vi "Acquire_Widefield.vi"() -> ()   [LabVIEW 2014]
uses:
  <vilib>/vision/Image Controls.llb/IMAQ Image.ctl
  <vilib>/userdefined/High Color/IMAQdx.ctl
  Widefield_globals.vi
  <vilib>/vision/NI_Vision_Development_Module.lvlib
  <vilib>/vision/driver/NI_Vision_Acquisition_Software.lvlib
panel:
  out "Camera Type":u16(ring)=1 items=["AVT Manta", "Hamamatsu Orca", "PhotonFocus GigE"]
  out "FOV size (um)":i32[](array[numeric])=[643, 394]
  in  "Spatial filter (um)":i32=100
  out "exposure (s)":dbl
  out "IMAQ session":T1 caption="Session Out"
  out "odor time":u32
  out "Waveform Graph":i32[](graph)
  out "frame gap":sgl
  out "frame times":i32[](array[numeric])
  out "error out":errorcluster
  out "LED settle":i32
  out "Control LED?":bool
  out "stim tag":string
  out "SF file":string
  out "One Bulb?":bool
  in  "Odor build up":dbl=5.0
  out "File Path":path
  out "SingleFrames":bool
  out "empty frame":dbl[][](array[numeric])
  out "Resolution":u32[](array[numeric])
  out "Experiment Sequence":dbl[][](array[numeric])
  out "settings":sgl[](array[numeric])
  out "Buff Img":T2
  out "IgorSAir":T2
  out "IgorOdor":T2
  out "IgorAir":T2
  out "RatioIm 2":dbl[][](graph)
  out "COString":string
  in  "Offset (32768 default)":u32=32768
  in  "Contrast \n(600000 default)":u32=600000
  out "FrameTime":u32
  in  "Pause":bool=TRUE
  out "ExpOrderRefnum":refnum<file>
  out "Subframes":u32
  out "DCSAir":dbl[][](array[numeric])
  out "DCOdor":dbl[][](array[numeric])
  out "DCAir":dbl[][](array[numeric])
  out "TiffRefnum":refnum<file>
  out "Indices":i32[](array[numeric])
  out "Frames SAir":u32
  out "RatioIm":dbl[][](graph)
  out "Odors:":u32
  out "StopAcq":bool
  in  "Stop":bool=TRUE
  out "Odor #":i32=50
  out "Repeats:":i32=1
  out "Repeat #":i32=1
  out "Frames Odor":u32
  out "Frames Air":u32
  out "Status":string
  out "Stimulus #":i32
  in  "start":bool=TRUE
  # "Filtered Ratio Image"
  # "Ratio Image"
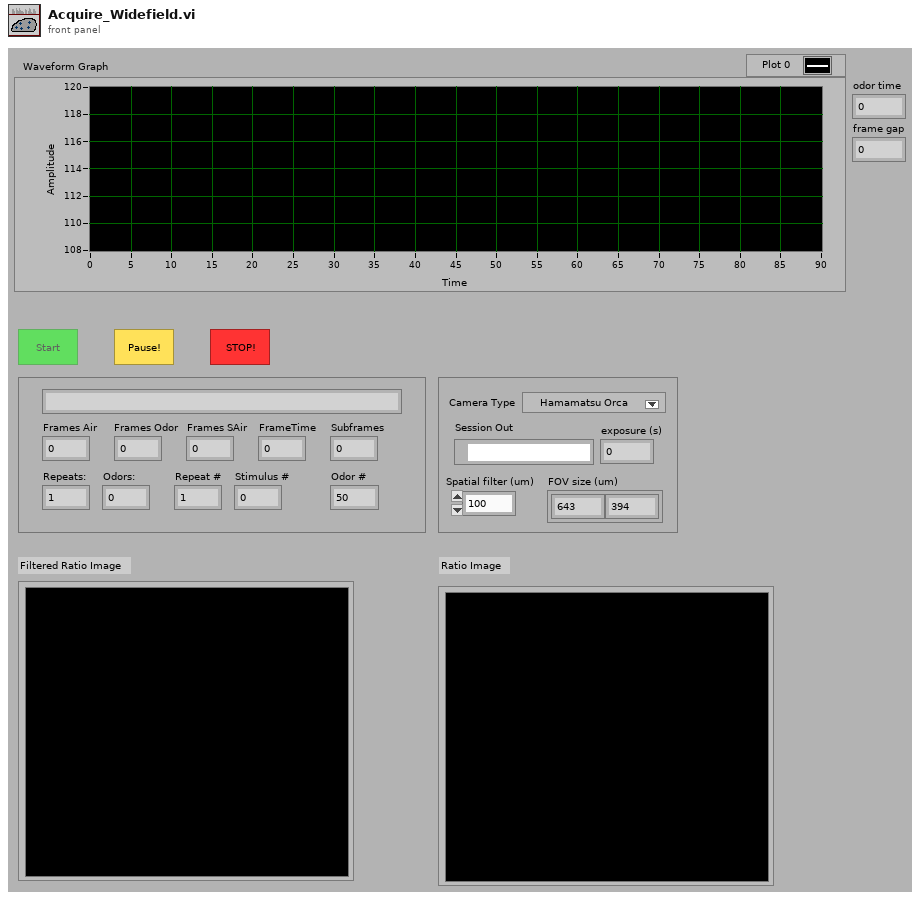
[diagram p1: front panel]
types:
  T1 = typedef "IMAQdx.ctl" = refnum<k21>
  T2 = typedef "IMAQ Image.ctl" = refnum<image>
  T3 = enum16{"open", "replace", "create", "open or create", "replace or create", "replace or create with confirmation"}
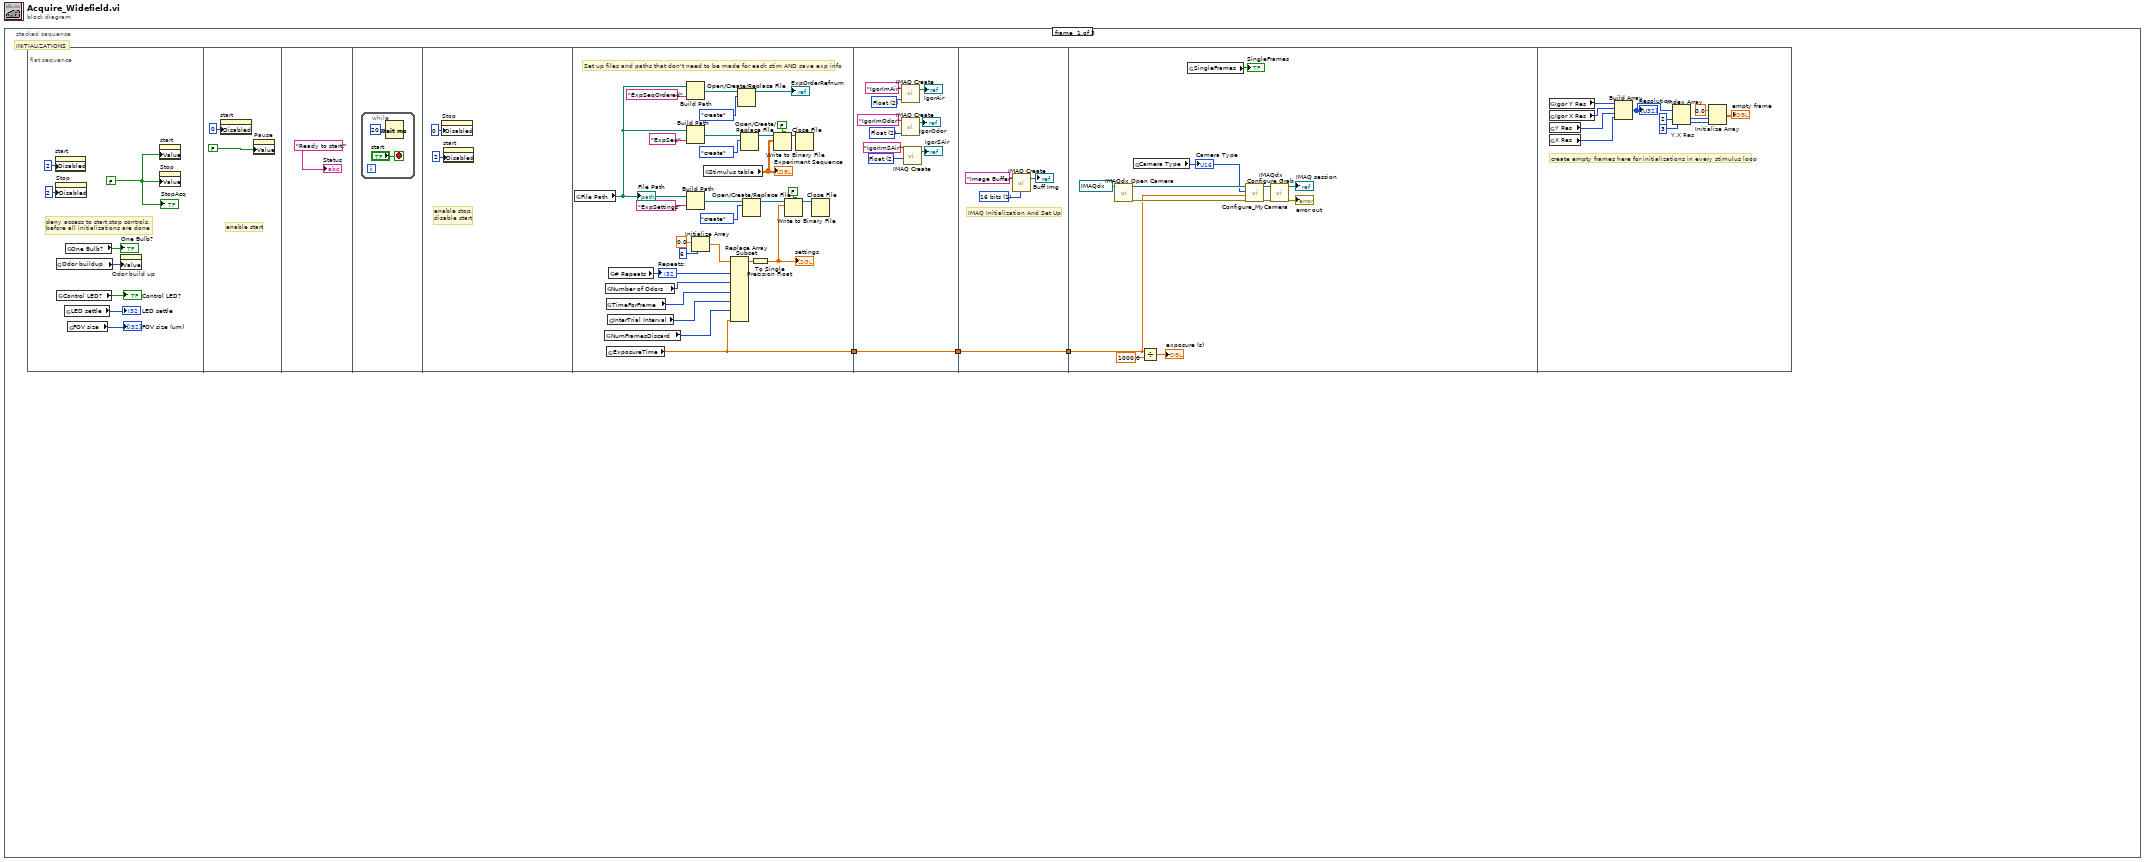
[diagram p0: block diagram]
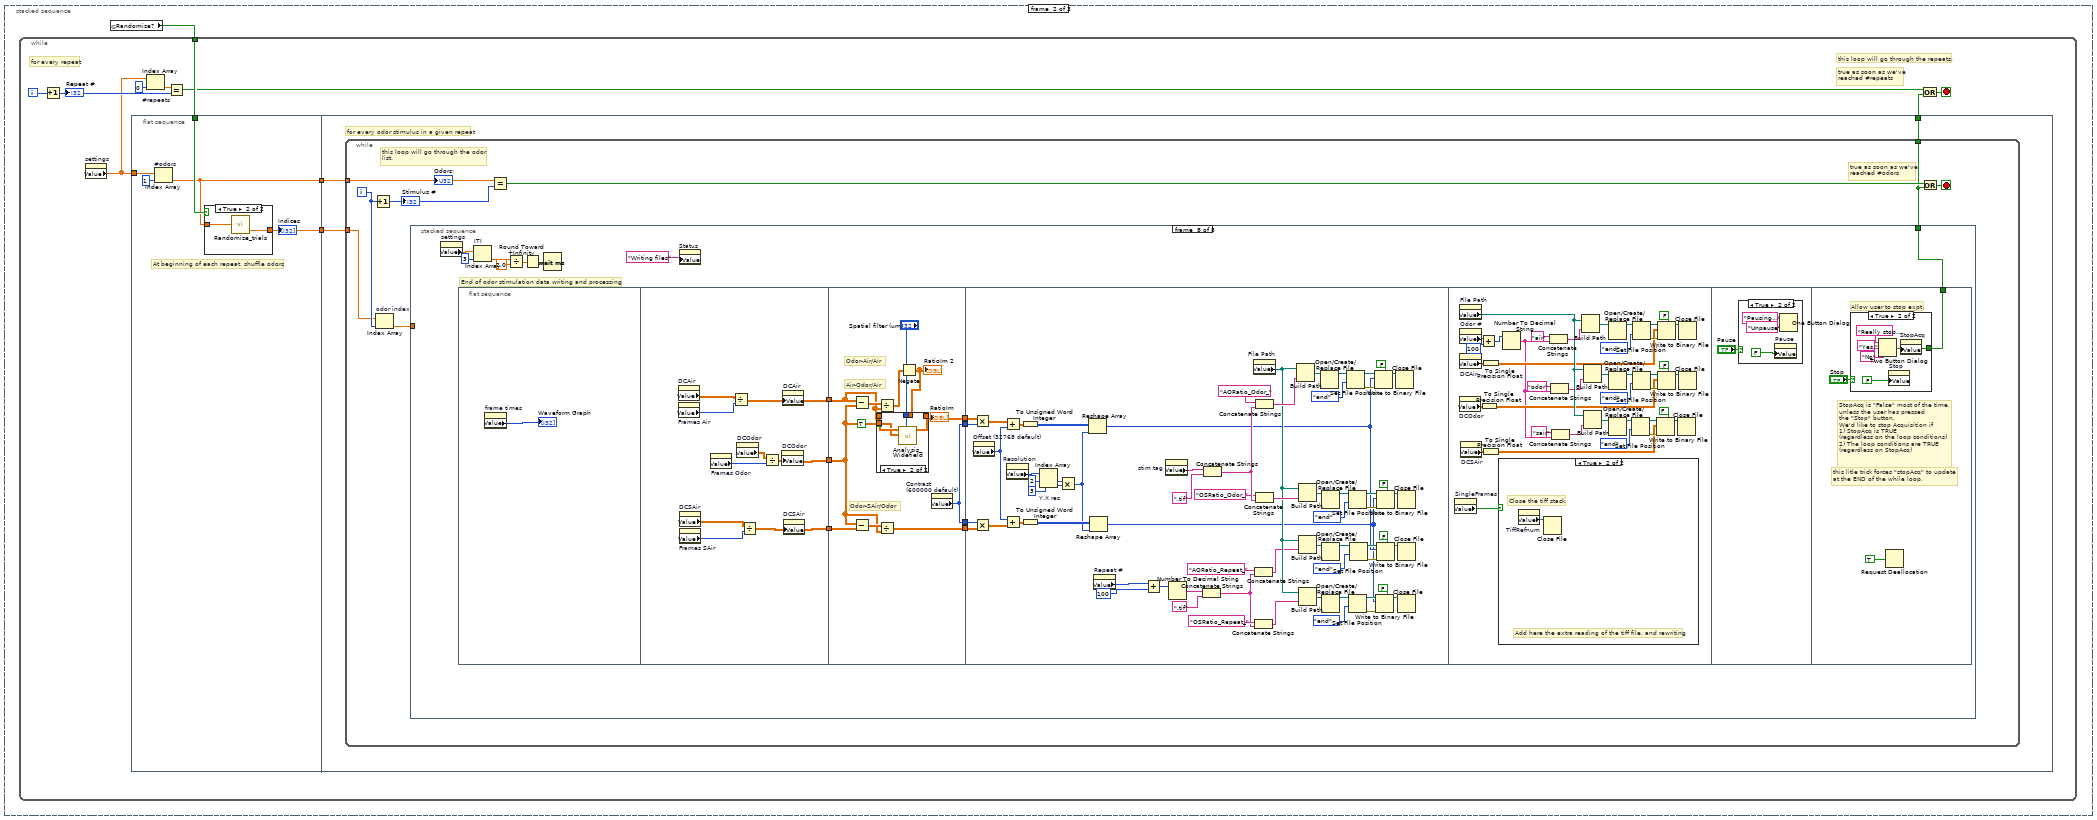
[diagram p2: hidden frame]
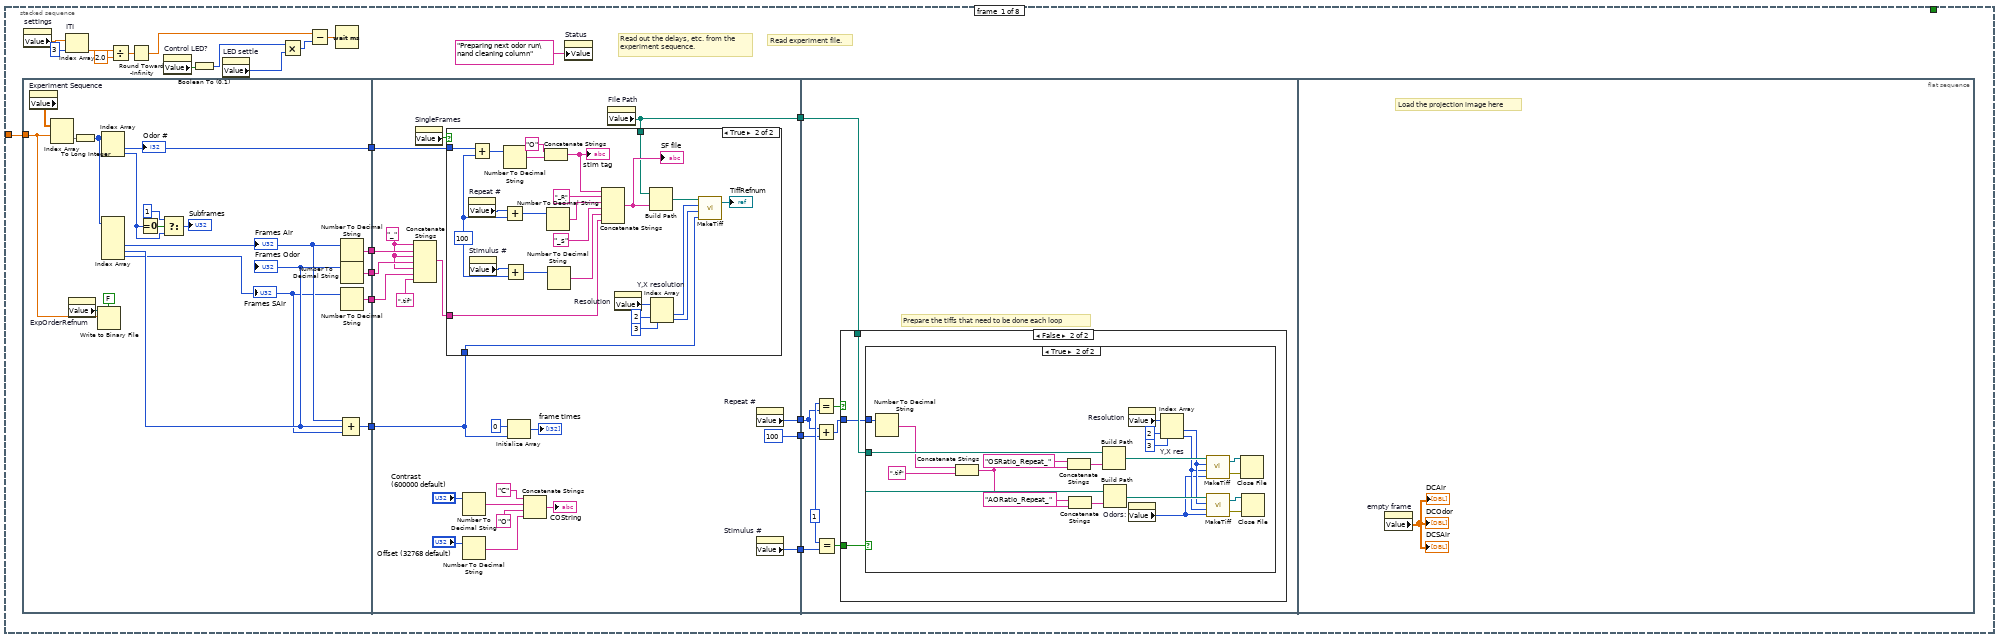
[diagram p4: hidden frame]
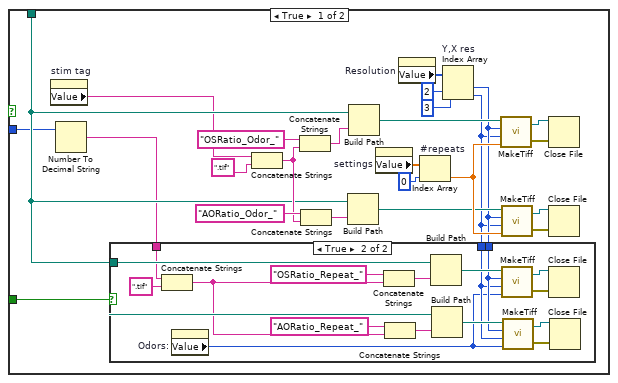
[diagram p6: hidden frame]
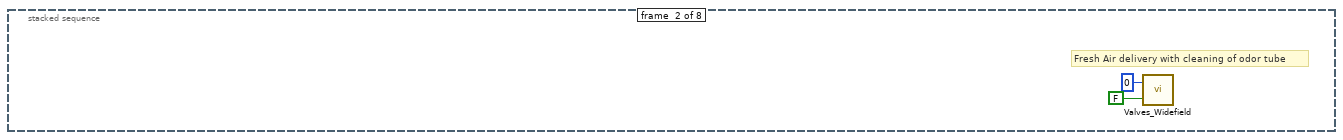
[diagram p9: hidden frame]
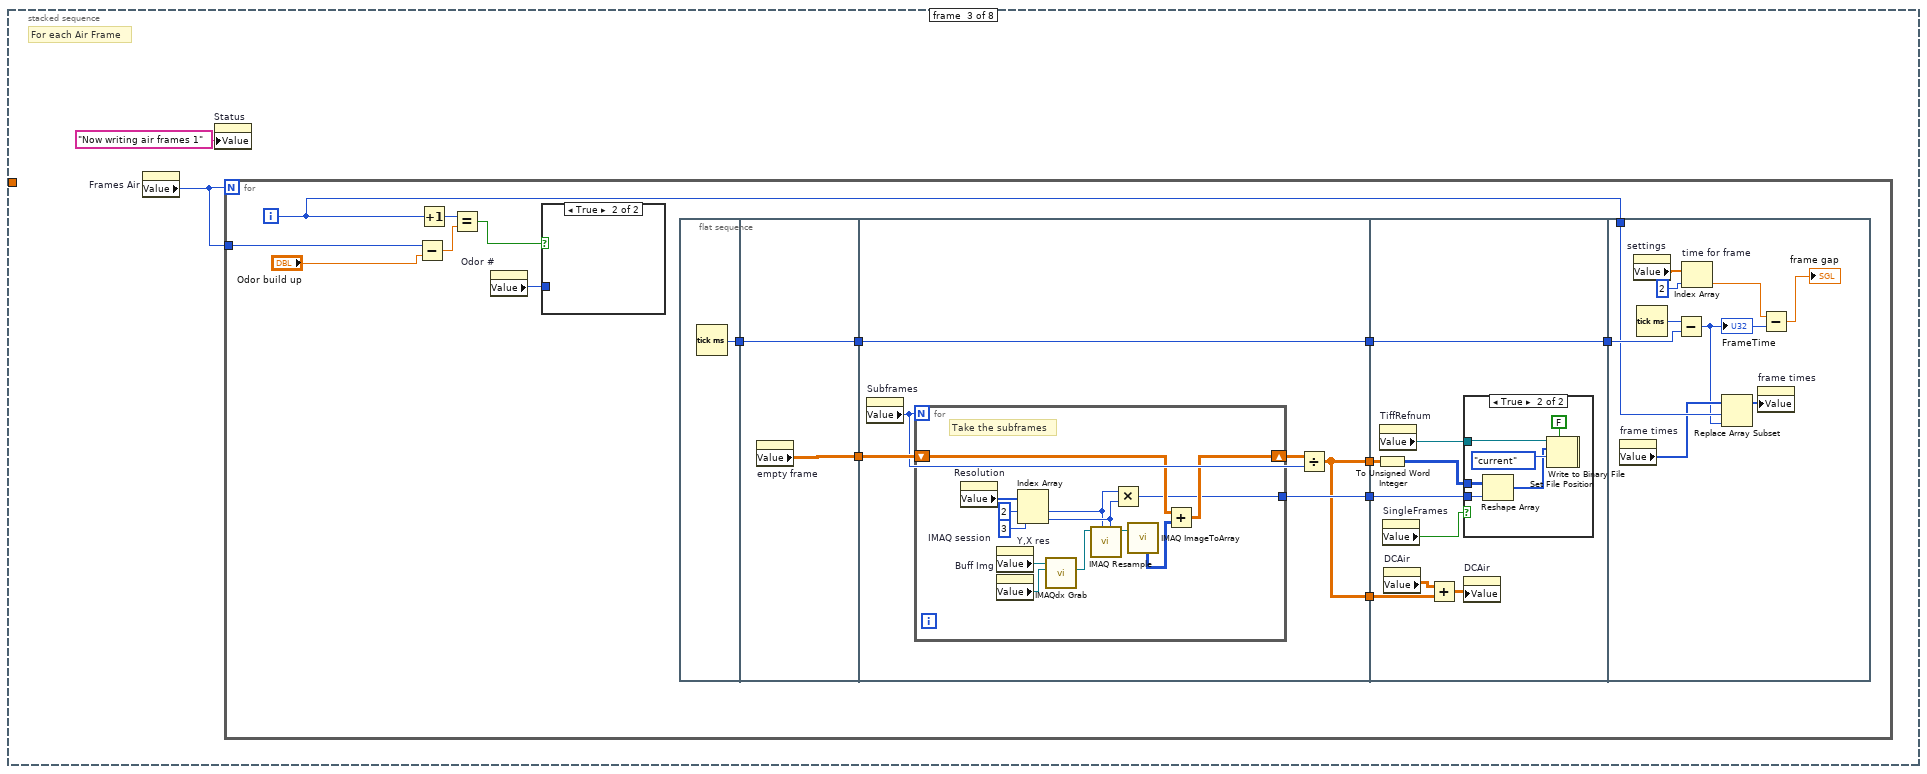
[diagram p10: hidden frame]
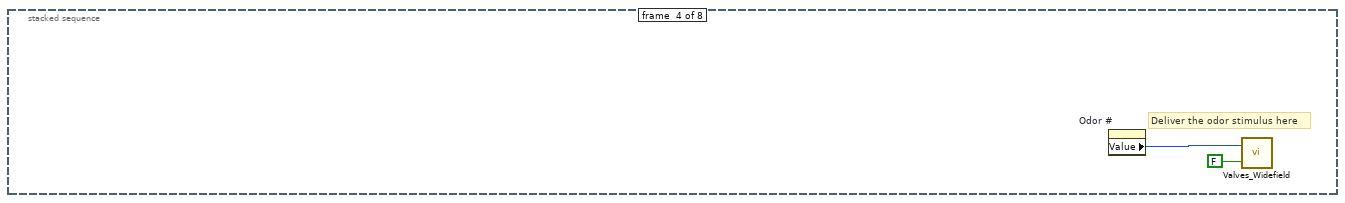
[diagram p13: hidden frame]
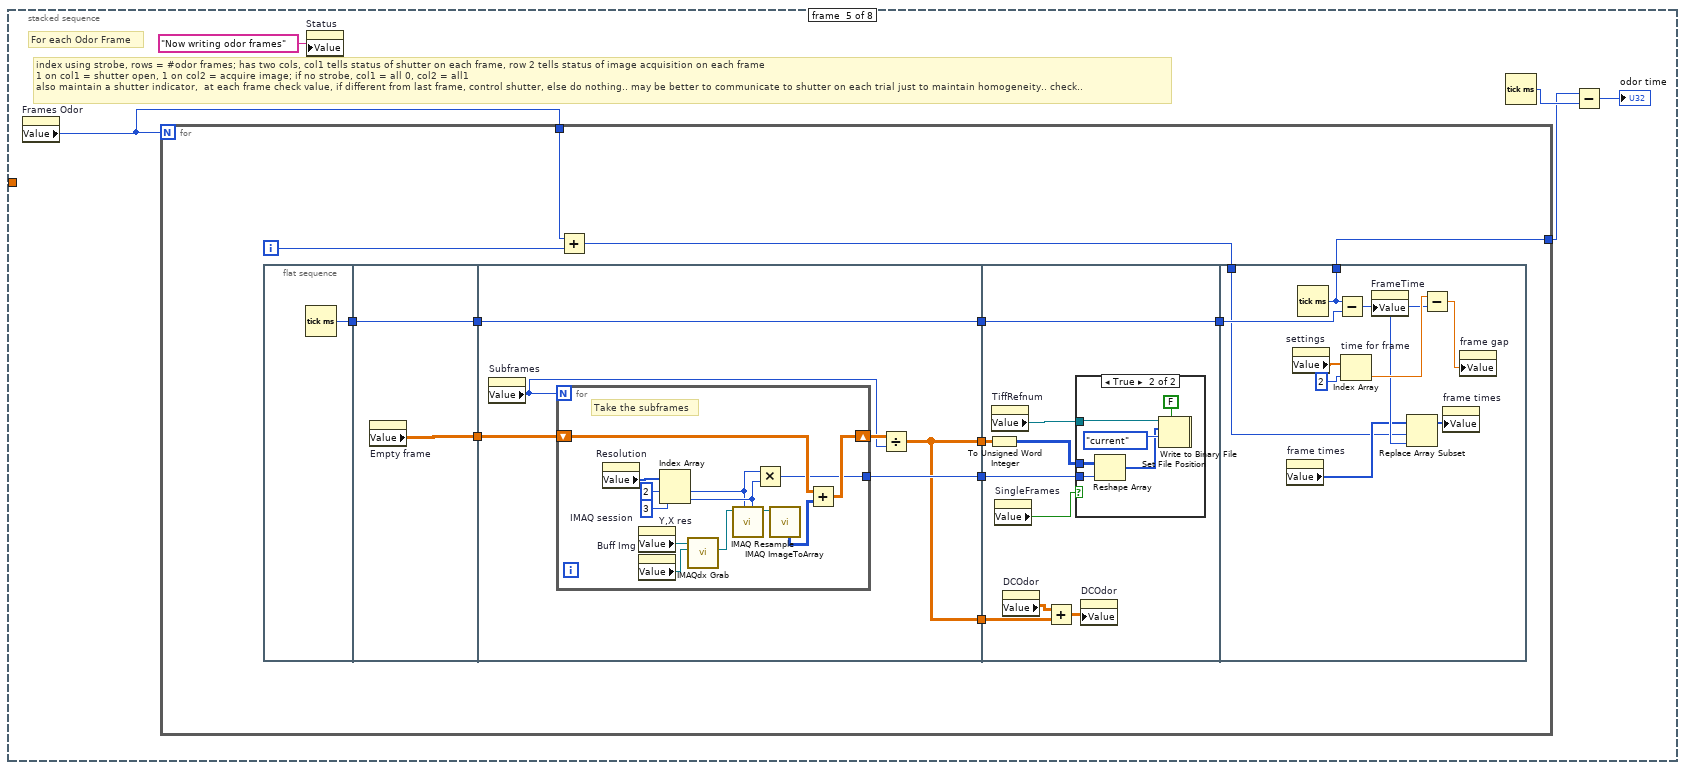
[diagram p14: hidden frame]
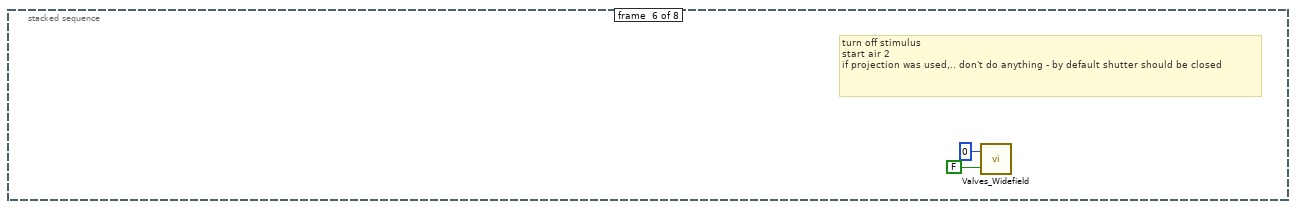
[diagram p16: hidden frame]
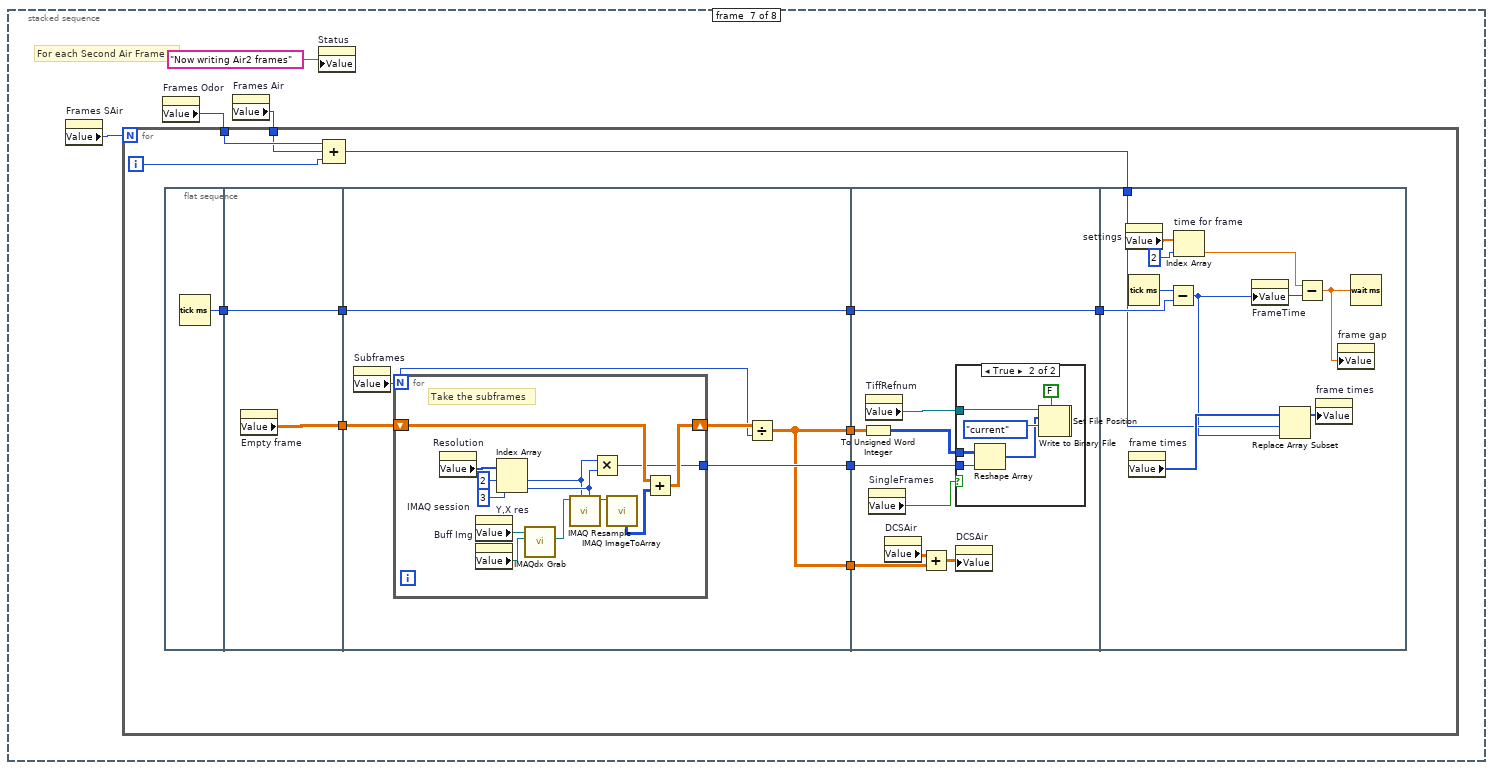
[diagram p17: hidden frame]
diagram:
  n1 = stacked-sequence {
    frame #0 {
      # "INITIALIZATIONS"
      n2 = flat-sequence {
        tunnel: [w20] -> w1
        tunnel: [w48] -> w2
        tunnel: w1 -> [w48]
        tunnel: [w58] -> w3
        tunnel: w2 -> [w58]
        tunnel: w3 -> [w65]
        frame #0 {
          w9 = FALSE ("Stop")
          # "deny access to start stop controls, \nbefore all initializations are done"
          n3 = property on="start" class="Bool (strict)"("Disabled"=u8 2) -> ()  [unwired: 2 in, 2 out]
          n4 = property on="Stop" class="Bool (strict)"("Disabled"=u8 2) -> ()  [unwired: 2 in, 2 out]
          n5 = global read "Widefield_globals.vi" "Odor buildup"() -> (w8:i32)
          n6 = global read "Widefield_globals.vi" "Control LED?"() -> (→"Control LED?":bool)
          n7 = global read "Widefield_globals.vi" "LED settle"() -> (→"LED settle":i32)
          n8 = global read "Widefield_globals.vi" "One Bulb?"() -> (→"One Bulb?":bool)
          n9 = global read "Widefield_globals.vi" "FOV size"() -> (→"FOV size (um)":i32[])
          n10 = property on="Odor build up" class="DigNum (strict)"("Value"=w8) -> ()  [unwired: 2 in, 2 out]
          n11 = property on="start" class="Bool (strict)"("Value"=w9) -> ()  [unwired: 2 in, 2 out]
          n12 = property on="Stop" class="Bool (strict)"("Value"=w9) -> ()  [unwired: 2 in, 2 out]
          "StopAcq" <- w9
        }
        frame #1 {
          # "enable start"
          n13 = property on="start" class="Bool (strict)"("Disabled"=u8 0) -> ()  [unwired: 2 in, 2 out]
          n14 = property on="Pause" class="Bool (strict)"("Value"=FALSE ("Pause")) -> ()  [unwired: 2 in, 2 out]
        }
        frame #2 {
          "Status" <- "Ready to start!" ("Status")
        }
        frame #3 {
          n15 = while {
            stop <- "start" stop-if-true
            n16 = Wait (ms)(milliseconds to wait=u32 20) -> ()  [unwired: 1 out]
          }
        }
        frame #4 {
          # "enable stop,\ndisable start"
          n17 = property on="Stop" class="Bool (strict)"("Disabled"=u8 0) -> ()  [unwired: 2 in, 2 out]
          n18 = property on="start" class="Bool (strict)"("Disabled"=u8 2) -> ()  [unwired: 2 in, 2 out]
        }
        frame #5 {
          # "Set up files and paths that don't need to be made for each stim AND save exp info"
          n19 = global read "Widefield_globals.vi" "File Path"() -> (w26:path)
          "File Path" <- w26
          n20 = global read "Widefield_globals.vi" "NumFramesDiscard"() -> (w21:i32)
          n21 = global read "Widefield_globals.vi" "Number of Odors"() -> (w23:u32)
          n22 = global read "Widefield_globals.vi" "TimeForFrame"() -> (w19:u32)
          n23 = global read "Widefield_globals.vi" "ExposureTime"() -> (w20:dbl)
          n24 = global read "Widefield_globals.vi" "InterTrial Interval"() -> (w22:i32)
          n25 = global read "Widefield_globals.vi" "# Repeats"() -> (w24:u16)
          "Repeats:" <- w24
          n26 = Build Path(base path=w26, name or relative path="ExpSeq" ("string")) -> (appended path=w39:path)
          n27 = Build Path(base path=w26, name or relative path="ExpSeqOrdered" ("string")) -> (appended path=w29:path)
          n28 = Build Path(base path=w26, name or relative path="ExpSettings" ("string")) -> (appended path=w37:path)
          n29 = Initialize Array(sgl 0.0 ("element"), 6 ("dimension size")) -> (w33:sgl[])
          n30 = global read "Widefield_globals.vi" "Stimulus table"() -> (w25:dbl[][])
          "Experiment Sequence" <- w25
          n31 = Replace Array Subset(array=w33, new element #1=w24, new element #2=w23, new element #3=w19, new element #4=w22, new element #5=w21, new element #6=w20) -> (w32:sgl[])  [unwired: 6 in]
          n32 = Open/Create/Replace File(file path (use dialog)=w29, operation (0:open)=T3."create") -> (refnum out=→"ExpOrderRefnum":refnum<file>)  [unwired: 1 in, 5 out]
          n33 = Open/Create/Replace File(file path (use dialog)=w39, operation (0:open)=T3."create") -> (refnum out=w46:refnum<file>)  [unwired: 1 in, 5 out]
          n34 = Open/Create/Replace File(file path (use dialog)=w37, operation (0:open)=T3."create") -> (refnum out=w45:refnum<file>)  [unwired: 1 in, 5 out]
          n35 = To Single Precision Float(number=w32) -> (single precision float=w31:sgl[])
          "settings" <- w31
          n36 = Write to Binary File(file (use dialog)=w46, data=w25, 5:FALSE ("prepend array or string size? (T)")) -> (refnum out=w47:refnum<file>)  [unwired: 1 in, 4 out]
          n37 = Write to Binary File(file (use dialog)=w45, data=w31, 5:FALSE ("prepend array or string size? (T)")) -> (refnum out=w30:refnum<file>)  [unwired: 1 in, 4 out]
          n38 = Close File(refnum=w47) -> ()  [unwired: 1 in, 2 out]
          n39 = Close File(refnum=w30) -> ()  [unwired: 1 in, 2 out]
        }
        frame #6 {
          w52 = u32 2 items=["8 bits", "16 bits", "Float", "Complex", "RGB", "HSL"] ("Image Type")
          w54 = u32 2 items=["8 bits", "16 bits", "Float", "Complex", "RGB", "HSL"] ("Image Type")
          w56 = u32 2 items=["8 bits", "16 bits", "Float", "Complex", "RGB", "HSL"] ("Image Type")
          n40 = call "IMAQ Create"("Image Name"="IgorImAir", "Image Type"=w56) -> ("New Image"=→"IgorAir":T2)  [unwired: 2 in, 2 out]
          n41 = call "IMAQ Create"("Image Name"="IgorImOdor", "Image Type"=w54) -> ("New Image"=→"IgorOdor":T2)  [unwired: 2 in, 2 out]
          n42 = call "IMAQ Create"("Image Name"="IgorImSAir", "Image Type"=w52) -> ("New Image"=→"IgorSAir":T2)  [unwired: 2 in, 2 out]
        }
        frame #7 {
          w61 = u32 1 items=["8 bits", "16 bits", "Float", "Complex", "RGB", "HSL"] ("Image Type")
          # "IMAQ Initialization And Set Up"
          n43 = call "IMAQ Create"("Image Name"="Image Buffer", "Image Type"=w61) -> ("New Image"=→"Buff Img":T2)  [unwired: 2 in, 2 out]
        }
        frame #8 {
          n44 = call <vilib>:"IMAQdx Open Camera.vi"("Session In"=T1 "cam0") -> ("error out"=w66:errorcluster, "Session Out"=w67:T1)  [unwired: 2 in, 7 out]
          n45 = global read "Widefield_globals.vi" "Camera Type"() -> (w62:u16)
          "Camera Type" <- w62
          n46 = Divide(x=w65, y=1000.0) -> (x/y=→"exposure (s)":dbl)
          n47 = global read "Widefield_globals.vi" "SingleFrames"() -> (→"SingleFrames":bool)
          n48 = call "Configure_MyCamera.vi"("Camera Error In"=w66, "ExposureTime (ms)"=w65, "Camera Type"=w62, "Camera Session In"=w67) -> ("Camera Error Out"=w63:errorcluster, "Camera Session Out"=w64:T1)  [unwired: 2 in]
          n49 = call <vilib>:"IMAQdx Configure Grab.vi"("error in"=w63, "Session In"=w64) -> ("error out"=→"error out":errorcluster, "Session Out"=→"IMAQ session":T1)  [unwired: 8 out]
        }
        frame #9 {
          # "create empty frames here for initializations in every stimulus loop"
          n50 = global read "Widefield_globals.vi" "Igor Y Res"() -> (w78:u32)
          n51 = global read "Widefield_globals.vi" "Igor X Res"() -> (w77:u32)
          n52 = global read "Widefield_globals.vi" "Y Res"() -> (w75:u32)
          n53 = global read "Widefield_globals.vi" "X Res"() -> (w74:u32)
          n54 = Build Array(w78, w77, w75, w74) -> (w76:u32[])
          "Resolution" <- w76
          n55 = Index Array "Y,X Res"(array=w76, index #1=2 ("index"), index #2=3 ("index")) -> (element #1=w84:u32, element #2=w83:u32)
          n56 = Initialize Array(0.0 ("element"), w84, w83) -> (→"empty frame":dbl[][])
        }
      }
    }
    frame #1 {
      n57 = global read "Widefield_globals.vi" "Randomize?"() -> (w85:bool)
      n58 = while {
        tunnel: w85 -> [w94]
        i -> [w89]
        stop <- w96 stop-if-true
        # "for every repeat"
        # "this loop will go through the repeats."
        # "true as soon as we've\nreached #repeats"
        n59 = Increment(x=w89) -> (x+1=w95:i32)
        "Repeat #" <- w95
        n60 = property on="settings" class="Arr (strict)"() -> ("Value"=w91:sgl[])  [unwired: 2 in, 2 out]
        n61 = flat-sequence {
          tunnel: w91 -> [w101]
          tunnel: w94 -> [w99]
          tunnel: [w98] -> w93
          tunnel: [w97] -> w92
          tunnel: w93 -> [w109]
          tunnel: w92 -> [w108]
          tunnel: [w107] -> w87
          frame #0 {
            # "At beginning of each repeat, shuffle odors"
            n62 = Index Array "#odors"(array=w101, index=1) -> (element=w98:sgl)
            n63 = case shown="True" w99 {
              tunnel: [w102 w106] -> w97
              tunnel: w98 -> [w103 w105]
              frame False {
                n64 = for {
                  N: w103 -> [_]
                  tunnel: [w104] -> w102 mode=indexing
                  i -> [w104]
                }
              }
              frame True {
                n65 = call "Randomize_trials.vi"("ArraySize"=w105) -> ("Randomized"=w106:dbl[])  [unwired: 2 in]
              }
            }
            "Indices" <- w97
          }
          frame #1 {
            # "for every odor stimulus in a given repeat"
            n66 = while {
              tunnel: w109 -> [w116]
              tunnel: w108 -> [w113]
              tunnel: [w111] -> w107
              i -> [w115]
              stop <- w117 stop-if-true
              # "this loop will go through the odor\nlist."
              # "true as soon as we've\nreached #odors"
              n67 = Increment(x=w115) -> (x+1=w110:i32)
              "Stimulus #" <- w110
              n68 = Index Array "odor index"(array=w113, index=w115) -> (element=w114:dbl)
              n69 = stacked-sequence {
                tunnel: w114 -> [w139 _ _ _ _ _ _ _]
                tunnel: [_ _ _ _ _ _ _ w490] -> w111
                frame #0 {
                  # "Read experiment file."
                  # "Read out the delays, etc. from the\nexperiment sequence."
                  n70 = flat-sequence {
                    tunnel: [w155] -> w138
                    tunnel: [w154] -> w137
                    tunnel: [w153] -> w136
                    tunnel: [w152] -> w135
                    tunnel: [w151] -> w134
                    tunnel: w139 -> [w143]
                    tunnel: [w171] -> w133
                    tunnel: [w172] -> w132
                    tunnel: [w170] -> w131
                    tunnel: w134 -> [w160]
                    tunnel: w135 -> [w166]
                    tunnel: w136 -> [w167]
                    tunnel: w137 -> [w168]
                    tunnel: w138 -> [w169]
                    tunnel: [100 ("y")] -> w123
                    tunnel: w133 -> [w206]
                    tunnel: w132 -> [w211]
                    tunnel: w131 -> [w210]
                    tunnel: w123 -> [w207]
                    frame #0 {
                      n71 = property on="Experiment Sequence" class="Arr (strict)"() -> ("Value"=w150:dbl[][])  [unwired: 2 in, 2 out]
                      n72 = Index Array(array=w150, index (row)=w143) -> (element=w149:dbl[])  [unwired: 1 in]
                      n73 = property on="ExpOrderRefnum" class="Ref (strict)"() -> ("Value"=w156:refnum<file>)  [unwired: 2 in, 2 out]
                      n74 = To Long Integer(number=w149) -> (32bit integer=w145:i32[])
                      n75 = Write to Binary File(file (use dialog)=w156, data=w143, 5:FALSE ("prepend array or string size? (T)")) -> ()  [unwired: 1 in, 5 out]
                      n76 = Index Array(array=w145) -> (element #1=w152:i32, element #2=w142:i32)  [unwired: 2 in]
                      "Odor #" <- w152
                      n77 = Index Array(array=w145) -> (element #3=w141:i32, element #4=w144:i32, element #5=w140:i32)  [unwired: 5 in, 2 out]
                      "Frames Air" <- w141
                      "Frames Odor" <- w144
                      "Frames SAir" <- w140
                      n78 = Equal To 0?(x=w142) -> (x = 0?=w148:bool)
                      n79 = Select(t=1, s=w148, f=w142) -> (s? t:f=→"Subframes":i32)
                      n80 = Number To Decimal String(number=w141) -> (decimal integer string=w155:string)  [unwired: 1 out]
                      n81 = Number To Decimal String(number=w144) -> (decimal integer string=w154:string)  [unwired: 1 out]
                      n82 = Number To Decimal String(number=w140) -> (decimal integer string=w153:string)  [unwired: 1 out]
                      n83 = Compound Arithmetic op=ADD(w141, w144, w140) -> (w151:i32)
                    }
                    frame #1 {
                      w163 = "_" ("string")
                      n84 = Concatenate Strings(w163, w169, w163, w168, w163, w167, ".tif" ("string")) -> (w164:string)
                      n85 = property on="SingleFrames" class="Bool (strict)"() -> ("Value"=w165:bool)  [unwired: 2 in, 2 out]
                      n86 = Number To Decimal String(number="Contrast \n(600000 default)") -> (decimal integer string=w175:string)  [unwired: 1 out]
                      n87 = Number To Decimal String(number="Offset (32768 default)") -> (decimal integer string=w174:string)  [unwired: 1 out]
                      n88 = Initialize Array(0 ("element"), w160) -> (→"frame times":i32[])
                      n89 = Concatenate Strings("C" ("string"), w175, "O" ("string"), w174) -> (→"COString":string)
                      n90 = property on="File Path" class="Path"() -> ("Value"=w172:path)  [unwired: 2 in, 2 out]
                      n91 = case shown="True" w165 {
                        tunnel: w166 -> [_ w199]
                        tunnel: w172 -> [_ w187]
                        tunnel: w164 -> [_ w180]
                        tunnel: w160 -> [_ w197]
                        frame False {
                        }
                        frame True {
                          w198 = 100 ("y")
                          n92 = property on="Repeat #" class="DigNum (strict)"() -> ("Value"=w190:i32)  [unwired: 2 in, 2 out]
                          n93 = property on="Stimulus #" class="DigNum (strict)"() -> ("Value"=w183:i32)  [unwired: 2 in, 2 out]
                          n94 = Add(x=w199, y=w198) -> (x+y=w203:i32)
                          n95 = Number To Decimal String(number=w203) -> (decimal integer string=w185:string)  [unwired: 1 out]
                          n96 = Add(x=w190, y=w198) -> (x+y=w204:i32)
                          n97 = Add(x=w183, y=w198) -> (x+y=w200:i32)
                          n98 = Concatenate Strings("O" ("string"), w185) -> (w184:string)
                          "stim tag" <- w184
                          n99 = Number To Decimal String(number=w204) -> (decimal integer string=w202:string)  [unwired: 1 out]
                          n100 = Number To Decimal String(number=w200) -> (decimal integer string=w181:string)  [unwired: 1 out]
                          n101 = Concatenate Strings(w184, "_R" ("string"), w202, "_s" ("string"), w181, w180) -> (w189:string)
                          "SF file" <- w189
                          n102 = property on="Resolution" class="Arr (strict)"() -> ("Value"=w195:u32[])  [unwired: 2 in, 2 out]
                          n103 = Build Path(base path=w187, name or relative path=w189) -> (appended path=w188:path)
                          n104 = Index Array "Y,X resolution"(array=w195, index #1=2 ("index"), index #2=3 ("index")) -> (element #1=w192:u32, element #2=w191:u32)
                          n105 = call "MakeTiff.vi"("z"=w197, "X"=w191, "Y"=w192, "file path"=w188) -> ("refnum tif"=→"TiffRefnum":refnum<file>)  [unwired: 1 out]
                        }
                      }
                      n106 = property on="Repeat #" class="DigNum (strict)"() -> ("Value"=w171:i32)  [unwired: 2 in, 2 out]
                      n107 = property on="Stimulus #" class="DigNum (strict)"() -> ("Value"=w170:i32)  [unwired: 2 in, 2 out]
                    }
                    frame #2 {
                      w209 = 1 ("x")
                      # "Prepare the tiffs that need to be done each loop"
                      n108 = Equal?(x=w209, y=w206) -> (x = y?=w212:bool)
                      n109 = Add(x=w206, y=w207) -> (x+y=w205:i32)
                      n110 = Equal?(x=w209, y=w210) -> (x = y?=w208:bool)
                      n111 = case shown="False" w212 {
                        tunnel: w211 -> [w220 w257]
                        tunnel: w205 -> [w216 w256]
                        tunnel: w208 -> [w215 w255]
                        frame True {
                          n112 = property on="stim tag" class="Str"() -> ("Value"=w214:string)  [unwired: 2 in, 2 out]
                          n113 = Number To Decimal String(number=w216) -> (decimal integer string=w217:string)  [unwired: 1 out]
                          n114 = Concatenate Strings(w214, ".tif" ("string")) -> (w229:string)
                          n115 = Concatenate Strings("OSRatio_Odor_" ("string"), w229) -> (w231:string)
                          n116 = Concatenate Strings("AORatio_Odor_" ("string"), w229) -> (w228:string)
                          n117 = Build Path(base path=w220, name or relative path=w228) -> (appended path=w221:path)
                          n118 = Build Path(base path=w220, name or relative path=w231) -> (appended path=w233:path)
                          n119 = property on="settings" class="Arr (strict)"() -> ("Value"=w223:sgl[])  [unwired: 2 in, 2 out]
                          n120 = property on="Resolution" class="Arr (strict)"() -> ("Value"=w227:u32[])  [unwired: 2 in, 2 out]
                          n121 = Index Array "#repeats"(array=w223, index=0) -> (element=w222:sgl)
                          n122 = Index Array "Y,X res"(array=w227, index #1=2 ("index"), index #2=3 ("index")) -> (element #1=w219:u32, element #2=w218:u32)
                          n123 = case shown="True" w215 {
                            tunnel: w220 -> [_ w244]
                            tunnel: w219 -> [_ w243]
                            tunnel: w218 -> [_ w242]
                            tunnel: w217 -> [_ w240]
                            frame False {
                            }
                            frame True {
                              n124 = Concatenate Strings(w240, ".tif" ("string")) -> (w241:string)
                              n125 = property on="Odors:" class="DigNum (strict)"() -> ("Value"=w239:u32)  [unwired: 2 in, 2 out]
                              n126 = Concatenate Strings("OSRatio_Repeat_" ("string"), w241) -> (w254:string)
                              n127 = Concatenate Strings("AORatio_Repeat_" ("string"), w241) -> (w246:string)
                              n128 = Build Path(base path=w244, name or relative path=w254) -> (appended path=w245:path)
                              n129 = Build Path(base path=w244, name or relative path=w246) -> (appended path=w248:path)
                              n130 = call "MakeTiff.vi"("z"=w239, "X"=w242, "Y"=w243, "file path"=w245) -> ("error out"=w252:errorcluster, "refnum tif"=w251:refnum<file>)
                              n131 = call "MakeTiff.vi"("z"=w239, "X"=w242, "Y"=w243, "file path"=w248) -> ("error out"=w249:errorcluster, "refnum tif"=w250:refnum<file>)
                              n132 = Close File(refnum=w251, error in=w252) -> ()  [unwired: 2 out]
                              n133 = Close File(refnum=w250, error in=w249) -> ()  [unwired: 2 out]
                            }
                          }
                          n134 = call "MakeTiff.vi"("z"=w222, "X"=w218, "Y"=w219, "file path"=w233) -> ("error out"=w234:errorcluster, "refnum tif"=w235:refnum<file>)
                          n135 = call "MakeTiff.vi"("z"=w222, "X"=w218, "Y"=w219, "file path"=w221) -> ("error out"=w236:errorcluster, "refnum tif"=w237:refnum<file>)
                          n136 = Close File(refnum=w235, error in=w234) -> ()  [unwired: 2 out]
                          n137 = Close File(refnum=w237, error in=w236) -> ()  [unwired: 2 out]
                        }
                        frame False {
                          n138 = case shown="True" w255 {
                            tunnel: w257 -> [_ w265]
                            tunnel: w256 -> [_ w260]
                            frame False {
                            }
                            frame True {
                              n139 = Number To Decimal String(number=w260) -> (decimal integer string=w261:string)  [unwired: 1 out]
                              n140 = Concatenate Strings(w261, ".tif" ("string")) -> (w262:string)
                              n141 = Concatenate Strings("OSRatio_Repeat_" ("string"), w262) -> (w275:string)
                              n142 = Concatenate Strings("AORatio_Repeat_" ("string"), w262) -> (w267:string)
                              n143 = Build Path(base path=w265, name or relative path=w275) -> (appended path=w266:path)
                              n144 = Build Path(base path=w265, name or relative path=w267) -> (appended path=w269:path)
                              n145 = property on="Resolution" class="Arr (strict)"() -> ("Value"=w278:u32[])  [unwired: 2 in, 2 out]
                              n146 = property on="Odors:" class="DigNum (strict)"() -> ("Value"=w259:u32)  [unwired: 2 in, 2 out]
                              n147 = Index Array "Y,X res"(array=w278, index #1=2 ("index"), index #2=3 ("index")) -> (element #1=w264:u32, element #2=w263:u32)
                              n148 = call "MakeTiff.vi"("z"=w259, "X"=w263, "Y"=w264, "file path"=w266) -> ("error out"=w273:errorcluster, "refnum tif"=w272:refnum<file>)
                              n149 = call "MakeTiff.vi"("z"=w259, "X"=w263, "Y"=w264, "file path"=w269) -> ("error out"=w270:errorcluster, "refnum tif"=w271:refnum<file>)
                              n150 = Close File(refnum=w272, error in=w273) -> ()  [unwired: 2 out]
                              n151 = Close File(refnum=w271, error in=w270) -> ()  [unwired: 2 out]
                            }
                          }
                        }
                      }
                    }
                    frame #3 {
                      # "Load the projection image here"
                      n152 = property on="empty frame" class="Arr (strict)"() -> ("Value"=→"DCAir" →"DCOdor" →"DCSAir":dbl[][])  [unwired: 2 in, 2 out]
                    }
                  }
                  n153 = property on="settings" class="Arr (strict)"() -> ("Value"=w130:sgl[])  [unwired: 2 in, 2 out]
                  n154 = Index Array "ITI"(array=w130, index=3) -> (element=w128:sgl)
                  n155 = Divide(x=w128, y=sgl 2.0) -> (x/y=w126:sgl)
                  n156 = Round Toward -Infinity(1:w126) -> (0:w125:sgl)
                  n157 = property on="Control LED?" class="Bool (strict)"() -> ("Value"=w121:bool)  [unwired: 2 in, 2 out]
                  n158 = Boolean To (0,1)(Boolean=w121) -> (0, 1=w119:i16)
                  n159 = property on="LED settle" class="DigNum (strict)"() -> ("Value"=w118:i32)  [unwired: 2 in, 2 out]
                  n160 = Multiply(x=w119, y=w118) -> (x*y=w120:i32)
                  n161 = Subtract(x=w125, y=w120) -> (x-y=w122:sgl)
                  n162 = Wait (ms)(milliseconds to wait=w122) -> ()  [unwired: 1 out]
                  n163 = property on="Status" class="Str"("Value"="Preparing next odor run\nand cleaning column" ("Status")) -> ()  [unwired: 2 in, 2 out]
                }
                frame #1 {
                  # "Fresh Air delivery with cleaning of odor tube"
                  n164 = call "Valves_Widefield.vi"("All Off?"=FALSE ("All off?"), "valve#"=0) -> ()  [unwired: 1 in]
                }
                frame #2 {
                  # "For each Air Frame"
                  n165 = property on="Frames Air" class="DigNum (strict)"() -> ("Value"=w283:u32)  [unwired: 2 in, 2 out]
                  n166 = property on="Status" class="Str"("Value"="Now writing air frames 1" ("String")) -> ()  [unwired: 2 in, 2 out]
                  n167 = for {
                    N: w283 -> [_]
                    tunnel: w283 -> [w296]
                    i -> [w286]
                    n168 = Subtract(x=w296, y="Odor build up") -> (x-y=w284:dbl)
                    n169 = Increment(x=w286) -> (x+1=w298:i32)
                    n170 = Equal?(x=w298, y=w284) -> (x = y?=w297:bool)
                    n171 = property on="Odor #" class="DigNum (strict)"() -> ("Value"=w295:i32)  [unwired: 2 in, 2 out]
                    n172 = case shown="True" w297 {
                      tunnel: w295 -> [_ _]
                      frame False {
                      }
                      frame True {
                      }
                    }
                    n173 = flat-sequence {
                      tunnel: [w299] -> w290
                      tunnel: [w300] -> w294
                      tunnel: w290 -> [w301]
                      tunnel: [w301] -> w289
                      tunnel: w294 -> [w307]
                      tunnel: [w304] -> w293
                      tunnel: [w303] -> w292
                      tunnel: [w303] -> w291
                      tunnel: w289 -> [w302]
                      tunnel: [w302] -> w288
                      tunnel: w293 -> [w329]
                      tunnel: w292 -> [w328]
                      tunnel: w291 -> [w322]
                      tunnel: w288 -> [w321]
                      tunnel: [w321] -> w287
                      tunnel: w287 -> [w342]
                      tunnel: w286 -> [w341]
                      frame #0 {
                        n174 = Tick Count (ms)() -> (millisecond timer value=w299:u32)
                      }
                      frame #1 {
                        n175 = property on="empty frame" class="Arr (strict)"() -> ("Value"=w300:dbl[][])  [unwired: 2 in, 2 out]
                      }
                      frame #2 {
                        n176 = property on="Subframes" class="DigNum (strict)"() -> ("Value"=w305:u32)  [unwired: 2 in, 2 out]
                        n177 = for {
                          N: w305 -> [_]
                          shift-right: [w315] -> w306
                          shift-left: w307 -> [w314]
                          tunnel: [w311] -> w304
                          # "Take the subframes"
                          n178 = property on="Resolution" class="Arr (strict)"() -> ("Value"=w318:u32[])  [unwired: 2 in, 2 out]
                          n179 = property on="IMAQ session" class="IMAQdx (strict)"() -> ("Value"=w316:T1)  [unwired: 2 in, 2 out]
                          n180 = property on="Buff Img" class="IMAQImage (strict)"() -> ("Value"=w317:T2)  [unwired: 2 in, 2 out]
                          n181 = Index Array "Y,X res"(array=w318, index #1=2 ("index"), index #2=3 ("index")) -> (element #1=w312:u32, element #2=w313:u32)
                          n182 = call <vilib>:"IMAQdx Grab.vi"("Image In"=w317, "Session In"=w316) -> ("Image Out"=w310:T2)  [unwired: 2 in, 7 out]
                          n183 = call "IMAQ Resample"("X Resolution"=w313, "Y Resolution"=w312, "Image Src"=w310) -> ("Image Dst Out"=w309:T2)  [unwired: 4 in, 4 out]
                          n184 = Multiply(x=w312, y=w313) -> (x*y=w311:u32)
                          n185 = call "IMAQ ImageToArray"("Image"=w309) -> ("Image Pixels (U16)"=w308:u16[][])  [unwired: 2 in, 5 out]
                          n186 = Add(x=w314, y=w308) -> (x+y=w315:dbl[][])
                        }
                        n187 = Divide(x=w306, y=w305) -> (x/y=w303:dbl[][])
                      }
                      frame #3 {
                        n188 = To Unsigned Word Integer(number=w328) -> (unsigned 16bit integer=w327:u16[][])
                        n189 = property on="TiffRefnum" class="Ref (strict)"() -> ("Value"=w326:refnum<file>)  [unwired: 2 in, 2 out]
                        n190 = property on="SingleFrames" class="Bool (strict)"() -> ("Value"=w325:bool)  [unwired: 2 in, 2 out]
                        n191 = property on="DCAir" class="Arr (strict)"() -> ("Value"=w323:dbl[][])  [unwired: 2 in, 2 out]
                        n192 = Add(x=w323, y=w322) -> (x+y=w324:dbl[][])
                        n193 = case shown="True" w325 {
                          tunnel: w329 -> [_ w336]
                          tunnel: w327 -> [_ w334]
                          tunnel: w326 -> [_ w333]
                          frame False {
                          }
                          frame True {
                            n194 = Reshape Array(w334, w336) -> (w335:u16[])
                            n195 = Set File Position(refnum=w333, from (0:start)=enum16{"start", "end", "current"}."current" ("pos mode (0:2)")) -> (refnum out=w332:refnum<file>, error out=w331:errorcluster)  [unwired: 1 in, 1 out]
                            n196 = Write to Binary File(file (use dialog)=w332, data=w335, error in=w331, 5:FALSE ("prepend array or string size? (T)")) -> ()  [unwired: 5 out]
                          }
                        }
                        n197 = property on="DCAir" class="Arr (strict)"("Value"=w324) -> ()  [unwired: 2 in, 2 out]
                      }
                      frame #4 {
                        n198 = property on="frame times" class="Arr (strict)"() -> ("Value"=w340:i32[])  [unwired: 2 in, 2 out]
                        n199 = property on="settings" class="Arr (strict)"() -> ("Value"=w346:sgl[])  [unwired: 2 in, 2 out]
                        n200 = Tick Count (ms)() -> (millisecond timer value=w343:u32)
                        n201 = Subtract(x=w343, y=w342) -> (x-y=w339:u32)
                        "FrameTime" <- w339
                        n202 = Index Array "time for frame"(array=w346, index=2) -> (element=w347:sgl)
                        n203 = Replace Array Subset(array=w340, new element=w339, index=w341) -> (w338:i32[])
                        n204 = property on="frame times" class="Arr (strict)"("Value"=w338) -> ()  [unwired: 2 in, 2 out]
                        n205 = Subtract(x=w347, y=w339) -> (x-y=→"frame gap":sgl)
                      }
                    }
                  }
                }
                frame #3 {
                  # "Deliver the odor stimulus here"
                  n206 = property on="Odor #" class="DigNum (strict)"() -> ("Value"=w348:i32)  [unwired: 2 in, 2 out]
                  n207 = call "Valves_Widefield.vi"("All Off?"=FALSE ("All off?"), "valve#"=w348) -> ()  [unwired: 1 in]
                }
                frame #4 {
                  # "index using strobe, rows = #odor frames; has two cols, col1 tells status of shutter on each frame, row 2 tells status of image acquisition on each frame\n1 on col1 = shutter open, 1 on col2 = acquire image; if no strobe, col1 = all 0, col2 = all1\nalso maintain a shutter indicator,  at each frame check value, if different from last frame, control shutter, else do nothing.. may be better to communicate to shutter on each trial just to maintain homogeneity.. check.."
                  # "For each Odor Frame"
                  n208 = property on="Frames Odor" class="DigNum (strict)"() -> ("Value"=w350:u32)  [unwired: 2 in, 2 out]
                  n209 = for {
                    N: w350 -> [_]
                    tunnel: w350 -> [w357]
                    tunnel: [w355] -> w351
                    i -> [w358]
                    n210 = flat-sequence {
                      tunnel: [w367] -> w366
                      tunnel: [w369] -> w365
                      tunnel: w366 -> [w368]
                      tunnel: [w368] -> w364
                      tunnel: w365 -> [w371]
                      tunnel: [w373] -> w363
                      tunnel: [w370] -> w362
                      tunnel: [w370] -> w361
                      tunnel: w364 -> [w372]
                      tunnel: [w372] -> w360
                      tunnel: w363 -> [w397]
                      tunnel: w362 -> [w396]
                      tunnel: w361 -> [w390]
                      tunnel: w360 -> [w389]
                      tunnel: [w389] -> w359
                      tunnel: w359 -> [w412]
                      tunnel: w356 -> [w408]
                      tunnel: [w406] -> w355
                      frame #0 {
                        n211 = Tick Count (ms)() -> (millisecond timer value=w367:u32)
                      }
                      frame #1 {
                        n212 = property on="Empty frame" class="Arr (strict)"() -> ("Value"=w369:dbl[][])  [unwired: 2 in, 2 out]
                      }
                      frame #2 {
                        n213 = property on="Subframes" class="DigNum (strict)"() -> ("Value"=w374:u32)  [unwired: 2 in, 2 out]
                        n214 = for {
                          N: w374 -> [_]
                          shift-right: [w381] -> w375
                          shift-left: w371 -> [w380]
                          tunnel: [w377] -> w373
                          # "Take the subframes"
                          n215 = property on="Resolution" class="Arr (strict)"() -> ("Value"=w384:u32[])  [unwired: 2 in, 2 out]
                          n216 = property on="IMAQ session" class="IMAQdx (strict)"() -> ("Value"=w382:T1)  [unwired: 2 in, 2 out]
                          n217 = property on="Buff Img" class="IMAQImage (strict)"() -> ("Value"=w383:T2)  [unwired: 2 in, 2 out]
                          n218 = Index Array "Y,X res"(array=w384, index #1=2 ("index"), index #2=3 ("index")) -> (element #1=w378:u32, element #2=w379:u32)
                          n219 = call <vilib>:"IMAQdx Grab.vi"("Image In"=w383, "Session In"=w382) -> ("Image Out"=w388:T2)  [unwired: 2 in, 7 out]
                          n220 = call "IMAQ Resample"("X Resolution"=w379, "Y Resolution"=w378, "Image Src"=w388) -> ("Image Dst Out"=w387:T2)  [unwired: 4 in, 4 out]
                          n221 = Multiply(x=w378, y=w379) -> (x*y=w377:u32)
                          n222 = call "IMAQ ImageToArray"("Image"=w387) -> ("Image Pixels (U16)"=w376:u16[][])  [unwired: 2 in, 5 out]
                          n223 = Add(x=w380, y=w376) -> (x+y=w381:dbl[][])
                        }
                        n224 = Divide(x=w375, y=w374) -> (x/y=w370:dbl[][])
                      }
                      frame #3 {
                        n225 = To Unsigned Word Integer(number=w396) -> (unsigned 16bit integer=w395:u16[][])
                        n226 = property on="TiffRefnum" class="Ref (strict)"() -> ("Value"=w394:refnum<file>)  [unwired: 2 in, 2 out]
                        n227 = property on="SingleFrames" class="Bool (strict)"() -> ("Value"=w393:bool)  [unwired: 2 in, 2 out]
                        n228 = property on="DCOdor" class="Arr (strict)"() -> ("Value"=w391:dbl[][])  [unwired: 2 in, 2 out]
                        n229 = Add(x=w391, y=w390) -> (x+y=w392:dbl[][])
                        n230 = case shown="True" w393 {
                          tunnel: w397 -> [_ w404]
                          tunnel: w395 -> [_ w402]
                          tunnel: w394 -> [_ w401]
                          frame False {
                          }
                          frame True {
                            n231 = Reshape Array(w402, w404) -> (w403:u16[])
                            n232 = Set File Position(refnum=w401, from (0:start)=enum16{"start", "end", "current"}."current" ("pos mode (0:2)")) -> (refnum out=w400:refnum<file>, error out=w399:errorcluster)  [unwired: 1 in, 1 out]
                            n233 = Write to Binary File(file (use dialog)=w400, data=w403, error in=w399, 5:FALSE ("prepend array or string size? (T)")) -> ()  [unwired: 5 out]
                          }
                        }
                        n234 = property on="DCOdor" class="Arr (strict)"("Value"=w392) -> ()  [unwired: 2 in, 2 out]
                      }
                      frame #4 {
                        n235 = property on="frame times" class="Arr (strict)"() -> ("Value"=w409:i32[])  [unwired: 2 in, 2 out]
                        n236 = property on="settings" class="Arr (strict)"() -> ("Value"=w414:sgl[])  [unwired: 2 in, 2 out]
                        n237 = Tick Count (ms)() -> (millisecond timer value=w406:u32)
                        n238 = Subtract(x=w406, y=w412) -> (x-y=w410:u32)
                        n239 = Index Array "time for frame"(array=w414, index=2) -> (element=w415:sgl)
                        n240 = property on="FrameTime" class="DigNum (strict)"("Value"=w410) -> ()  [unwired: 2 in, 2 out]
                        n241 = Replace Array Subset(array=w409, new element=w410, index=w408) -> (w411:i32[])
                        n242 = Subtract(x=w415, y=w410) -> (x-y=w407:sgl)
                        n243 = property on="frame times" class="Arr (strict)"("Value"=w411) -> ()  [unwired: 2 in, 2 out]
                        n244 = property on="frame gap" class="DigNum (strict)"("Value"=w407) -> ()  [unwired: 2 in, 2 out]
                      }
                    }
                    n245 = Add(x=w357, y=w358) -> (x+y=w356:u32)
                  }
                  n246 = property on="Status" class="Str"("Value"="Now writing odor frames" ("String")) -> ()  [unwired: 2 in, 2 out]
                  n247 = Tick Count (ms)() -> (millisecond timer value=w352:u32)
                  n248 = Subtract(x=w351, y=w352) -> (x-y=→"odor time":u32)
                }
                frame #5 {
                  # "turn off stimulus\nstart air 2\nif projection was used,.. don't do anything - by default shutter should be closed"
                  n249 = call "Valves_Widefield.vi"("All Off?"=FALSE ("All off?"), "valve#"=0) -> ()  [unwired: 1 in]
                }
                frame #6 {
                  # "For each Second Air Frame"
                  n250 = property on="Frames SAir" class="DigNum (strict)"() -> ("Value"=w420:u32)  [unwired: 2 in, 2 out]
                  n251 = property on="Frames Odor" class="DigNum (strict)"() -> ("Value"=w418:u32)  [unwired: 2 in, 2 out]
                  n252 = property on="Frames Air" class="DigNum (strict)"() -> ("Value"=w419:u32)  [unwired: 2 in, 2 out]
                  n253 = for {
                    N: w420 -> [_]
                    tunnel: w418 -> [w425]
                    tunnel: w419 -> [w422]
                    i -> [w424]
                    n254 = flat-sequence {
                      tunnel: [w434] -> w433
                      tunnel: [w436] -> w432
                      tunnel: w433 -> [w435]
                      tunnel: [w435] -> w431
                      tunnel: w432 -> [w442]
                      tunnel: [w439] -> w430
                      tunnel: [w437] -> w429
                      tunnel: [w437] -> w428
                      tunnel: w431 -> [w438]
                      tunnel: [w438] -> w427
                      tunnel: w430 -> [w464]
                      tunnel: w429 -> [w463]
                      tunnel: w428 -> [w457]
                      tunnel: w427 -> [w456]
                      tunnel: [w456] -> w426
                      tunnel: w426 -> [w478]
                      tunnel: w423 -> [w474]
                      frame #0 {
                        n255 = Tick Count (ms)() -> (millisecond timer value=w434:u32)
                      }
                      frame #1 {
                        n256 = property on="Empty frame" class="Arr (strict)"() -> ("Value"=w436:dbl[][])  [unwired: 2 in, 2 out]
                      }
                      frame #2 {
                        n257 = property on="Subframes" class="DigNum (strict)"() -> ("Value"=w440:u32)  [unwired: 2 in, 2 out]
                        n258 = for {
                          N: w440 -> [_]
                          shift-right: [w448] -> w441
                          shift-left: w442 -> [w447]
                          tunnel: [w444] -> w439
                          # "Take the subframes"
                          n259 = property on="Resolution" class="Arr (strict)"() -> ("Value"=w451:u32[])  [unwired: 2 in, 2 out]
                          n260 = property on="IMAQ session" class="IMAQdx (strict)"() -> ("Value"=w449:T1)  [unwired: 2 in, 2 out]
                          n261 = property on="Buff Img" class="IMAQImage (strict)"() -> ("Value"=w450:T2)  [unwired: 2 in, 2 out]
                          n262 = Index Array "Y,X res"(array=w451, index #1=2 ("index"), index #2=3 ("index")) -> (element #1=w445:u32, element #2=w446:u32)
                          n263 = call <vilib>:"IMAQdx Grab.vi"("Image In"=w450, "Session In"=w449) -> ("Image Out"=w455:T2)  [unwired: 2 in, 7 out]
                          n264 = call "IMAQ Resample"("X Resolution"=w446, "Y Resolution"=w445, "Image Src"=w455) -> ("Image Dst Out"=w454:T2)  [unwired: 4 in, 4 out]
                          n265 = Multiply(x=w445, y=w446) -> (x*y=w444:u32)
                          n266 = call "IMAQ ImageToArray"("Image"=w454) -> ("Image Pixels (U16)"=w443:u16[][])  [unwired: 2 in, 5 out]
                          n267 = Add(x=w447, y=w443) -> (x+y=w448:dbl[][])
                        }
                        n268 = Divide(x=w441, y=w440) -> (x/y=w437:dbl[][])
                      }
                      frame #3 {
                        n269 = To Unsigned Word Integer(number=w463) -> (unsigned 16bit integer=w462:u16[][])
                        n270 = property on="TiffRefnum" class="Ref (strict)"() -> ("Value"=w461:refnum<file>)  [unwired: 2 in, 2 out]
                        n271 = property on="SingleFrames" class="Bool (strict)"() -> ("Value"=w460:bool)  [unwired: 2 in, 2 out]
                        n272 = property on="DCSAir" class="Arr (strict)"() -> ("Value"=w458:dbl[][])  [unwired: 2 in, 2 out]
                        n273 = Add(x=w458, y=w457) -> (x+y=w459:dbl[][])
                        n274 = case shown="True" w460 {
                          tunnel: w464 -> [_ w471]
                          tunnel: w462 -> [_ w469]
                          tunnel: w461 -> [_ w468]
                          frame False {
                          }
                          frame True {
                            n275 = Reshape Array(w469, w471) -> (w470:u16[])
                            n276 = Set File Position(refnum=w468, from (0:start)=enum16{"start", "end", "current"}."current" ("pos mode (0:2)")) -> (refnum out=w467:refnum<file>, error out=w466:errorcluster)  [unwired: 1 in, 1 out]
                            n277 = Write to Binary File(file (use dialog)=w467, data=w470, error in=w466, 5:FALSE ("prepend array or string size? (T)")) -> ()  [unwired: 5 out]
                          }
                        }
                        n278 = property on="DCSAir" class="Arr (strict)"("Value"=w459) -> ()  [unwired: 2 in, 2 out]
                      }
                      frame #4 {
                        n279 = property on="settings" class="Arr (strict)"() -> ("Value"=w481:sgl[])  [unwired: 2 in, 2 out]
                        n280 = Tick Count (ms)() -> (millisecond timer value=w479:u32)
                        n281 = property on="frame times" class="Arr (strict)"() -> ("Value"=w476:i32[])  [unwired: 2 in, 2 out]
                        n282 = Subtract(x=w479, y=w478) -> (x-y=w473:u32)
                        n283 = Index Array "time for frame"(array=w481, index=2) -> (element=w482:sgl)
                        n284 = property on="FrameTime" class="DigNum (strict)"("Value"=w473) -> ()  [unwired: 2 in, 2 out]
                        n285 = Replace Array Subset(array=w476, new element=w473, index=w474) -> (w475:i32[])
                        n286 = Subtract(x=w482, y=w473) -> (x-y=w477:sgl)
                        n287 = property on="frame times" class="Arr (strict)"("Value"=w475) -> ()  [unwired: 2 in, 2 out]
                        n288 = property on="frame gap" class="DigNum (strict)"("Value"=w477) -> ()  [unwired: 2 in, 2 out]
                        n289 = Wait (ms)(milliseconds to wait=w477) -> ()  [unwired: 1 out]
                      }
                    }
                    n290 = Compound Arithmetic op=ADD(w425, w422, w424) -> (w423:u32)
                  }
                  n291 = property on="Status" class="Str"("Value"="Now writing Air2 frames" ("String")) -> ()  [unwired: 2 in, 2 out]
                }
                frame #7 {
                  # "End of odor stimulation data writing and processing"
                  n292 = property on="settings" class="Arr (strict)"() -> ("Value"=w489:sgl[])  [unwired: 2 in, 2 out]
                  n293 = flat-sequence {
                    tunnel: [w507] -> w497
                    tunnel: [w501] -> w496
                    tunnel: [w504] -> w495
                    tunnel: w497 -> [w518]
                    tunnel: w496 -> [w514]
                    tunnel: w495 -> [w515]
                    tunnel: [w513] -> w494
                    tunnel: [w512] -> w493
                    tunnel: [w511] -> w492
                    tunnel: [w511] -> w491
                    tunnel: w494 -> [w589]
                    tunnel: w493 -> [w588]
                    tunnel: w492 -> [w587]
                    tunnel: w491 -> [w586]
                    tunnel: [w635] -> w490
                    frame #0 {
                      n294 = property on="frame times" class="Arr (strict)"() -> ("Value"=→"Waveform Graph":i32[])  [unwired: 2 in, 2 out]
                    }
                    frame #1 {
                      n295 = property on="DCAir" class="Arr (strict)"() -> ("Value"=w499:dbl[][])  [unwired: 2 in, 2 out]
                      n296 = property on="Frames Air" class="DigNum (strict)"() -> ("Value"=w502:u32)  [unwired: 2 in, 2 out]
                      n297 = property on="DCSAir" class="Arr (strict)"() -> ("Value"=w505:dbl[][])  [unwired: 2 in, 2 out]
                      n298 = property on="Frames SAir" class="DigNum (strict)"() -> ("Value"=w503:u32)  [unwired: 2 in, 2 out]
                      n299 = property on="Frames Odor" class="DigNum (strict)"() -> ("Value"=w500:u32)  [unwired: 2 in, 2 out]
                      n300 = Divide(x=w499, y=w502) -> (x/y=w507:dbl[][])
                      n301 = property on="DCOdor" class="Arr (strict)"() -> ("Value"=w506:dbl[][])  [unwired: 2 in, 2 out]
                      n302 = Divide(x=w505, y=w503) -> (x/y=w504:dbl[][])
                      n303 = Divide(x=w506, y=w500) -> (x/y=w501:dbl[][])
                      n304 = property on="DCOdor" class="Arr (strict)"("Value"=w501) -> ()  [unwired: 2 in, 2 out]
                      n305 = property on="DCAir" class="Arr (strict)"("Value"=w507) -> ()  [unwired: 2 in, 2 out]
                      n306 = property on="DCSAir" class="Arr (strict)"("Value"=w504) -> ()  [unwired: 2 in, 2 out]
                    }
                    frame #2 {
                      # "Odor-SAir/Odor"
                      # "Odor-Air/Air"
                      # "Air-Odor/Air"
                      n307 = Subtract(x=w518, y=w514) -> (x-y=w519:dbl[][])
                      n308 = Subtract(x=w514, y=w515) -> (x-y=w516:dbl[][])
                      n309 = Divide(x=w519, y=w518) -> (x/y=w517:dbl[][])
                      n310 = Divide(x=w516, y=w514) -> (x/y=w512:dbl[][])
                      n311 = Negate(x=w517) -> (-x=w509:dbl[][])
                      "RatioIm 2" <- w509
                      n312 = case shown="True" TRUE {
                        tunnel: w518 -> [_ w524]
                        tunnel: w514 -> [_ w523]
                        tunnel: [w520 w522] -> w513
                        tunnel: w509 -> [w520 _]
                        tunnel: "Spatial filter (um)" -> [_ w521]
                        frame False {
                        }
                        frame True {
                          n313 = call "Analysis_Widefield.vi"("Spatial filter size (um)"=w521, "Image_odor"=w523, "Image_air"=w524) -> ("single precision float"=w522:sgl[][])  [unwired: 5 in, 1 out]
                        }
                      }
                      "RatioIm" <- w513
                      n314 = property on="Contrast \n(600000 default)" class="DigNum (strict)"() -> ("Value"=w511:u32)  [unwired: 2 in, 2 out]
                    }
                    frame #3 {
                      n315 = property on="Offset (32768 default)" class="DigNum (strict)"() -> ("Value"=w583:u32)  [unwired: 2 in, 2 out]
                      n316 = Multiply(x=w589, y=w587) -> (x*y=w585:dbl[][])
                      n317 = Multiply(x=w586, y=w588) -> (x*y=w584:dbl[][])
                      n318 = Add(x=w585, y=w583) -> (x+y=w582:dbl[][])
                      n319 = Add(x=w583, y=w584) -> (x+y=w581:dbl[][])
                      n320 = property on="Resolution" class="Arr (strict)"() -> ("Value"=w576:u32[])  [unwired: 2 in, 2 out]
                      n321 = To Unsigned Word Integer(number=w582) -> (unsigned 16bit integer=w580:u16[][])
                      n322 = To Unsigned Word Integer(number=w581) -> (unsigned 16bit integer=w579:u16[][])
                      n323 = Index Array "Y,X res"(array=w576, index #1=2 ("index"), index #2=3 ("index")) -> (element #1=w577:u32, element #2=w578:u32)
                      n324 = Multiply(x=w577, y=w578) -> (x*y=w573:u32)
                      n325 = Reshape Array(w580, w573) -> (w530:u16[])
                      n326 = Reshape Array(w579, w573) -> (w529:u16[])
                      n327 = property on="Repeat #" class="DigNum (strict)"() -> ("Value"=w550:i32)  [unwired: 2 in, 2 out]
                      n328 = Add(x=w550, y=100) -> (x+y=w527:i32)
                      n329 = property on="stim tag" class="Str"() -> ("Value"=w528:string)  [unwired: 2 in, 2 out]
                      n330 = Number To Decimal String(number=w527) -> (decimal integer string=w551:string)  [unwired: 1 out]
                      n331 = Concatenate Strings(w551, ".tif" ("string")) -> (w548:string)
                      n332 = Concatenate Strings(w528, ".tif" ("string")) -> (w570:string)
                      n333 = property on="File Path" class="Path"() -> ("Value"=w533:path)  [unwired: 2 in, 2 out]
                      n334 = Concatenate Strings("AORatio_Repeat_" ("string"), w548) -> (w531:string)
                      n335 = Concatenate Strings("OSRatio_Repeat_" ("string"), w548) -> (w532:string)
                      n336 = Concatenate Strings("OSRatio_Odor_" ("string"), w570) -> (w553:string)
                      n337 = Concatenate Strings("AORatio_Odor_" ("string"), w570) -> (w554:string)
                      n338 = Build Path(base path=w533, name or relative path=w554) -> (appended path=w561:path)
                      n339 = Build Path(base path=w533, name or relative path=w532) -> (appended path=w534:path)
                      n340 = Build Path(base path=w533, name or relative path=w553) -> (appended path=w562:path)
                      n341 = Build Path(base path=w533, name or relative path=w531) -> (appended path=w547:path)
                      n342 = Open/Create/Replace File(file path (use dialog)=w561) -> (refnum out=w556:refnum<file>)  [unwired: 1 in, 6 out]
                      n343 = Open/Create/Replace File(file path (use dialog)=w534) -> (refnum out=w539:refnum<file>)  [unwired: 1 in, 6 out]
                      n344 = Open/Create/Replace File(file path (use dialog)=w562) -> (refnum out=w567:refnum<file>)  [unwired: 1 in, 6 out]
                      n345 = Open/Create/Replace File(file path (use dialog)=w547) -> (refnum out=w542:refnum<file>)  [unwired: 1 in, 6 out]
                      n346 = Set File Position(refnum=w556, from (0:start)=enum16{"start", "end", "current"}."end" ("pos mode (0:2)")) -> (refnum out=w558:refnum<file>, error out=w559:errorcluster)  [unwired: 1 in, 1 out]
                      n347 = Set File Position(refnum=w567, from (0:start)=enum16{"start", "end", "current"}."end" ("pos mode (0:2)")) -> (refnum out=w565:refnum<file>, error out=w564:errorcluster)  [unwired: 2 in]
                      n348 = Set File Position(refnum=w539, from (0:start)=enum16{"start", "end", "current"}."end" ("pos mode (0:2)")) -> (refnum out=w537:refnum<file>, error out=w536:errorcluster)  [unwired: 2 in]
                      n349 = Set File Position(refnum=w542, from (0:start)=enum16{"start", "end", "current"}."end" ("pos mode (0:2)")) -> (refnum out=w544:refnum<file>, error out=w545:errorcluster)  [unwired: 2 in]
                      n350 = Write to Binary File(file (use dialog)=w558, data=w530, error in=w559, 5:FALSE ("prepend array or string size? (T)")) -> (refnum out=w557:refnum<file>)  [unwired: 4 out]
                      n351 = Write to Binary File(file (use dialog)=w537, data=w529, error in=w536, 5:FALSE ("prepend array or string size? (T)")) -> (refnum out=w538:refnum<file>)  [unwired: 4 out]
                      n352 = Write to Binary File(file (use dialog)=w565, data=w529, error in=w564, 5:FALSE ("prepend array or string size? (T)")) -> (refnum out=w566:refnum<file>)  [unwired: 4 out]
                      n353 = Write to Binary File(file (use dialog)=w544, data=w530, error in=w545, 5:FALSE ("prepend array or string size? (T)")) -> (refnum out=w543:refnum<file>)  [unwired: 1 in, 3 out]
                      n354 = Close File(refnum=w557) -> ()  [unwired: 1 in, 2 out]
                      n355 = Close File(refnum=w538) -> ()  [unwired: 1 in, 2 out]
                      n356 = Close File(refnum=w566) -> ()  [unwired: 1 in, 2 out]
                      n357 = Close File(refnum=w543) -> ()  [unwired: 1 in, 2 out]
                    }
                    frame #4 {
                      n358 = property on="SingleFrames" class="Bool (strict)"() -> ("Value"=w592:bool)  [unwired: 2 in, 2 out]
                      n359 = property on="DCOdor" class="Arr (strict)"() -> ("Value"=w627:dbl[][])  [unwired: 2 in, 2 out]
                      n360 = property on="File Path" class="Path"() -> ("Value"=w625:path)  [unwired: 2 in, 2 out]
                      n361 = property on="Odor #" class="DigNum (strict)"() -> ("Value"=w618:i32)  [unwired: 2 in, 2 out]
                      n362 = property on="DCAir" class="Arr (strict)"() -> ("Value"=w628:dbl[][])  [unwired: 2 in, 2 out]
                      n363 = property on="DCSAir" class="Arr (strict)"() -> ("Value"=w626:dbl[][])  [unwired: 2 in, 2 out]
                      n364 = Add(x=w618, y=100) -> (x+y=w591:i32)
                      n365 = To Single Precision Float(number=w627) -> (single precision float=w601:sgl[][])
                      n366 = To Single Precision Float(number=w628) -> (single precision float=w602:sgl[][])
                      n367 = To Single Precision Float(number=w626) -> (single precision float=w600:sgl[][])
                      n368 = case shown="True" w592 {
                        frame False {
                        }
                        frame True {
                          # "Add here the extra reading of the tiff file, and rewriting"
                          # "Close the tiff stack"
                          n369 = property on="TiffRefnum" class="Ref (strict)"() -> ("Value"=w629:refnum<file>)  [unwired: 2 in, 2 out]
                          n370 = Close File(refnum=w629) -> ()  [unwired: 1 in, 2 out]
                        }
                      }
                      n371 = Number To Decimal String(number=w591) -> (decimal integer string=w593:string)  [unwired: 1 out]
                      n372 = Concatenate Strings("air" ("string"), w593) -> (w598:string)
                      n373 = Concatenate Strings("odor" ("string"), w593) -> (w597:string)
                      n374 = Concatenate Strings("sair" ("string"), w593) -> (w594:string)
                      n375 = Build Path(base path=w625, name or relative path=w598) -> (appended path=w603:path)
                      n376 = Build Path(base path=w625, name or relative path=w597) -> (appended path=w604:path)
                      n377 = Build Path(base path=w625, name or relative path=w594) -> (appended path=w605:path)
                      n378 = Open/Create/Replace File(file path (use dialog)=w605) -> (refnum out=w607:refnum<file>)  [unwired: 1 in, 6 out]
                      n379 = Open/Create/Replace File(file path (use dialog)=w603) -> (refnum out=w620:refnum<file>)  [unwired: 1 in, 6 out]
                      n380 = Open/Create/Replace File(file path (use dialog)=w604) -> (refnum out=w616:refnum<file>)  [unwired: 1 in, 6 out]
                      n381 = Set File Position(refnum=w607, from (0:start)=enum16{"start", "end", "current"}."end" ("pos mode (0:2)")) -> (refnum out=w609:refnum<file>, error out=w610:errorcluster)  [unwired: 1 in, 1 out]
                      n382 = Set File Position(refnum=w620, from (0:start)=enum16{"start", "end", "current"}."end" ("pos mode (0:2)")) -> (refnum out=w622:refnum<file>, error out=w623:errorcluster)  [unwired: 1 in, 1 out]
                      n383 = Set File Position(refnum=w616, from (0:start)=enum16{"start", "end", "current"}."end" ("pos mode (0:2)")) -> (refnum out=w614:refnum<file>, error out=w613:errorcluster)  [unwired: 1 in, 1 out]
                      n384 = Write to Binary File(file (use dialog)=w609, data=w600, error in=w610, 5:FALSE ("prepend array or string size? (T)")) -> (refnum out=w608:refnum<file>)  [unwired: 4 out]
                      n385 = Write to Binary File(file (use dialog)=w622, data=w602, error in=w623, 5:FALSE ("prepend array or string size? (T)")) -> (refnum out=w621:refnum<file>)  [unwired: 4 out]
                      n386 = Write to Binary File(file (use dialog)=w614, data=w601, error in=w613, 5:FALSE ("prepend array or string size? (T)")) -> (refnum out=w615:refnum<file>)  [unwired: 4 out]
                      n387 = Close File(refnum=w608) -> ()  [unwired: 1 in, 2 out]
                      n388 = Close File(refnum=w621) -> ()  [unwired: 1 in, 2 out]
                      n389 = Close File(refnum=w615) -> ()  [unwired: 1 in, 2 out]
                    }
                    frame #5 {
                      n390 = case shown="True" "Pause" {
                        frame False {
                        }
                        frame True {
                          n391 = property on="Pause" class="Bool (strict)"("Value"=FALSE ("Pause")) -> ()  [unwired: 2 in, 2 out]
                          n392 = One Button Dialog(message="Pausing...", button name ("OK")="Unpause") -> ()  [unwired: 1 out]
                        }
                      }
                    }
                    frame #6 {
                      # "this litle trick forces \"stopAcq\" to update\nat the END of the while loop."
                      # "StopAcq is \"False\" most of the time, \nunless the user has pressed\nthe \"Stop\" button.\nWe'd like to stop Acquisition if\n1) StopAcq is TRUE \n(regardless on the loop conditions)\n2) The loop conditions are TRUE \n(regardless on StopAcq)"
                      # "Allow user to stop expt."
                      n393 = case shown="True" "Stop" {
                        tunnel: [w637 w638] -> w635
                        frame False {
                          n394 = property on="StopAcq" class="Bool (strict)"() -> ("Value"=w637:bool)  [unwired: 2 in, 2 out]
                        }
                        frame True {
                          n395 = Two Button Dialog(message="Really stop acquisition after this stimulus?", 1:"No" ("F button name (\"Cancel\")"), 2:"Yes." ("T button name (\"OK\")")) -> (T button?=w638:bool)
                          n396 = property on="Stop" class="Bool (strict)"("Value"=FALSE ("Stop")) -> ()  [unwired: 2 in, 2 out]
                          n397 = property on="StopAcq" class="Bool (strict)"("Value"=w638) -> ()  [unwired: 2 in, 2 out]
                        }
                      }
                      n398 = Request Deallocation(TRUE ("flag")) -> ()
                    }
                  }
                  n399 = Index Array "ITI"(array=w489, index=3) -> (element=w487:sgl)
                  n400 = Divide(x=w487, y=sgl 2.0) -> (x/y=w485:sgl)
                  n401 = Round Toward +Infinity(x=w485) -> (ceil(x): smallest int >= x=w484:sgl)
                  n402 = Wait (ms)(milliseconds to wait=w484) -> ()  [unwired: 1 out]
                  n403 = property on="Status" class="Str"("Value"="Writing files" ("String")) -> ()  [unwired: 2 in, 2 out]
                }
              }
              n404 = Equal?(x=w116, y=w110) -> (x = y?=w112:bool)
              n405 = Or(x=w112, y=w111) -> (x .or. y?=w117:bool)
              "Odors:" <- w116
            }
          }
        }
        n406 = Index Array "#repeats"(array=w91, index=0) -> (element=w90:sgl)
        n407 = Equal?(x=w90, y=w95) -> (x = y?=w88:bool)
        n408 = Or(x=w88, y=w87) -> (x .or. y?=w96:bool)
      }
    }
    frame #2 {
      n409 = property on="ExpOrderRefnum" class="Ref (strict)"() -> ("Value"=w645:refnum<file>)  [unwired: 2 in, 2 out]
      n410 = property on="Status" class="Str"("Value"="Done!" ("Status")) -> ()  [unwired: 2 in, 2 out]
      n411 = property on="StopAcq" class="Bool (strict)"("Value"=TRUE ("StopAcq")) -> ()  [unwired: 2 in, 2 out]
      n412 = property on="IMAQ session" class="IMAQdx (strict)"() -> ("Value"=w643:T1)  [unwired: 2 in, 2 out]
      n413 = call <vilib>:"IMAQdx Close Camera.vi"("Session In"=w643) -> ()  [unwired: 1 in, 10 out]
      n414 = Close File(refnum=w645) -> ()  [unwired: 1 in, 2 out]
    }
  }
